vi "Read Terminals and Acyclic Frame Names.vi"(8 "error in":errorcluster, 11 "port":T1 format="%.0x") -> (0 "error out":errorcluster, 1 "terminal names":string[](array[string]), 2 "terminals":T2[](array[typedef]), 3 "port out":T1 format="%.0x", 4 "acyclic frame names":string[](array[string]))   [LabVIEW 2020, in "AIM MIL-STD-1553 Scripting.lvlib"]
doc: "Returns a <b>terminal name</b> and <b>terminal address</b> for each terminal in the <b>port</b>. Also returns the <b>acyclic frame names</b> from the Bus Controller within the psort."
uses:
  AIM MIL-STD-1553 Scripting.lvlib
  Shared/Address.ctl
  <vilib>/NI VeriStand/Custom Device API/Custom Device Item Ref.ctl
  Constants.vi
  <vilib>/NI VeriStand/Custom Device Tools/Custom Device Utility Library/NI VeriStand - Search for All Items by GUID.vi
  <vilib>/NI VeriStand/Custom Device API/Get Item Property (String).vi
  <vilib>/NI VeriStand/Custom Device Tools/Custom Device Utility Library/Custom Device Utility Library.lvlib
  <vilib>/NI VeriStand/Custom Device API/Custom Device API.lvlib
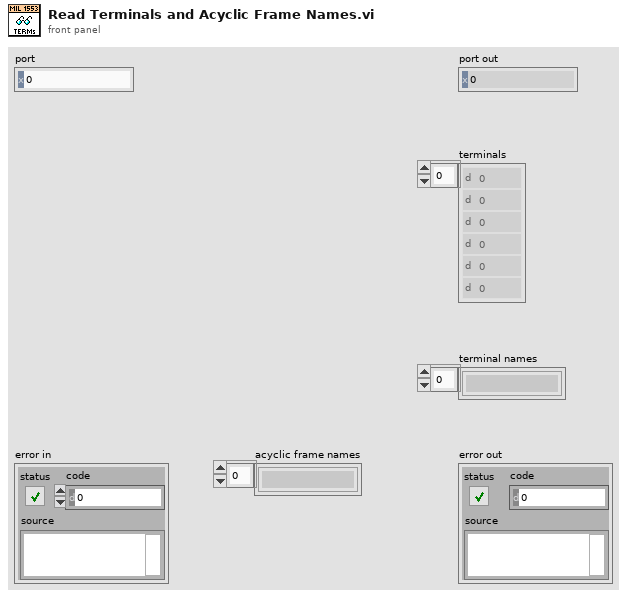
[diagram p1: front panel]
types:
  T1 = typedef "Custom Device API.lvlib/Custom Device Item Ref.ctl" = u64
  T2 = typedef "Address.ctl" = u16
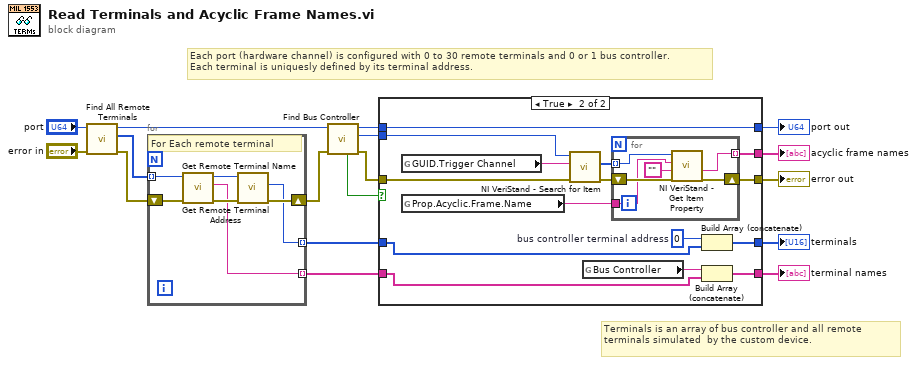
[diagram p0: block diagram]
diagram:
  # "Terminals is an array of bus controller and all remote terminals simulated  by the custom device."
  # "Each port (hardware channel) is configured with 0 to 30 remote terminals and 0 or 1 bus controller. \nEach terminal is uniquesly defined by its terminal address."
  n1 = call "Find All Remote Terminals.vi"("error in"="error in", "port"="port") -> ("error out"=w8:errorcluster, "remote terminals"=w10:T1[], "port out"=w13:T1)  [unwired: 7 in]
  n2 = for {
    shift-right: [w24] -> w14
    shift-left: w8 -> [w20]
    tunnel: w10 -> [w21] mode=indexing
    tunnel: [w23] -> w2 mode=indexing
    tunnel: [w18] -> w1 mode=indexing
    # "For Each remote terminal"
    n3 = call "Get Remote Terminal Name.vi"("error in"=w20, "remote terminal"=w21) -> ("error out"=w19:errorcluster, "terminal name"=w18:string, "remote terminal out"=w22:T1)  [unwired: 7 in]
    n4 = call "Get Remote Terminal Address.vi"("error in"=w19, "remote terminal"=w22) -> ("error out"=w24:errorcluster, "terminal address"=w23:T2)  [unwired: 6 in, 2 out]
  }
  n5 = call "Find Bus Controller.vi"("error in"=w14, "port"=w13) -> ("error out"=w7:errorcluster, "bus controller"=w9:T1, "port out"=w5:T1, "found?"=w6:bool)  [unwired: 6 in]
  n6 = case shown="True" w6 {
    tunnel: w5 -> [w28 w43]
    tunnel: w7 -> [w27 w39]
    tunnel: [w28 w43] -> w4
    tunnel: [w27 w35] -> w16
    tunnel: w9 -> [_ w41]
    tunnel: [w25 w42] -> w15
    tunnel: [_ w34] -> w17
    tunnel: [w26 w31] -> w3
    tunnel: w2 -> [w25 w30]
    tunnel: w1 -> [w26 w29]
    frame False {
    }
    frame True {
      w33 = T2 0  # bus controller terminal address
      n7 = global read "Constants.vi" "GUID.Trigger Channel"() -> (w40:string)
      n8 = global read "Constants.vi" "Prop.Acyclic.Frame.Name"() -> (w36:string)
      n9 = call-poly <vilib>:"NI VeriStand - Search for Item.vi"("error in"=w39, "Item GUID"=w40, "Section Ref in"=w41) -> ("error out"=w37:errorcluster, "Item Refs"=w38:T1[])  [unwired: 5 in, 2 out]
      n10 = global read "Constants.vi" "Bus Controller"() -> (w32:string)
      n11 = for {
        tunnel: w38 -> [w48] mode=indexing
        shift-right: [w49] -> w35
        shift-left: w37 -> [w47]
        tunnel: w36 -> [w46]
        tunnel: [w44] -> w34 mode=indexing
        n12 = call-poly <vilib>:"NI VeriStand - Get Item Property.vi"("error in (no error)"=w47, "Default Value"="", "Property Name"=w46, "Item Ref in"=w48) -> ("error out"=w49:errorcluster, "Value"=w44:string)  [unwired: 4 in, 2 out]
      }
      n13 = Build Array (concatenate)(w33, w30) -> (w42:T2[])
      n14 = Build Array (concatenate)(w32, w29) -> (w31:string[])
    }
  }
  "acyclic frame names" <- w17
  "error out" <- w16
  "terminals" <- w15
  "port out" <- w4
  "terminal names" <- w3
